vi "test Add Find Remove CD.vi"(8 "error in (no error)":errorcluster, 11 "TestCase in":refnum<class "Embedded Data Logger Scripting Unit Tests.lvclass">) -> (0 "error out":errorcluster, 3 "TestCase out":refnum<class "Embedded Data Logger Scripting Unit Tests.lvclass">)   [LabVIEW 2027, in "Embedded Data Logger Scripting Unit Tests.lvclass"]
uses:
  Embedded Data Logger Scripting Unit Tests.lvclass
  C:/Program Files/National Instruments/LabVIEW 2027/vi.lib/NI/VeriStand Custom Device Testing Tools/VeriStandScriptingTestCase/VeriStandScriptingTestCase.lvclass
  <vilib>/NI VeriStand/Custom Device API/Custom Device Item Ref.ctl
  <vilib>/NI/VeriStand Custom Device Testing Tools/VeriStandScriptingTestCase/VeriStandScriptingTestCase.lvclass/VeriStandScriptingTestCase.ctl
  <vilib>/NI/VeriStand Custom Device Testing Tools/VeriStandScriptingTestCase/Read Target.vi
  C:/NetCoreDLL/NationalInstruments.VeriStand.SystemDefinitionAPI.dll
  NetCoreDLL/NationalInstruments.VeriStand.SystemDefinitionAPI.dll
  C:/Program Files/National Instruments/LabVIEW 2027/vi.lib/addons/_JKI Toolkits/VI Tester/TestCase.llb/TestCase.lvclass
  <vilib>/addons/_JKI Toolkits/VI Tester/TestCase.llb/TestCase.lvclass
  Embedded Data Logger Scripting.lvlib
  <vilib>/NI VeriStand/Custom Device API/Custom Device API.lvlib
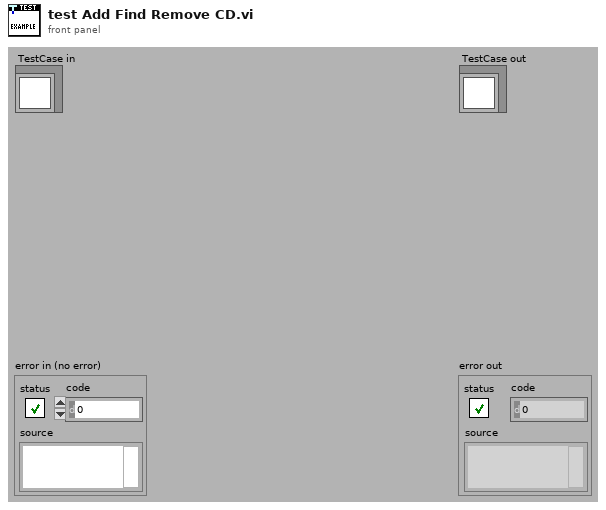
[diagram p1: front panel]
types:
  T1 = typedef "Custom Device API.lvlib/Custom Device Item Ref.ctl" = u64
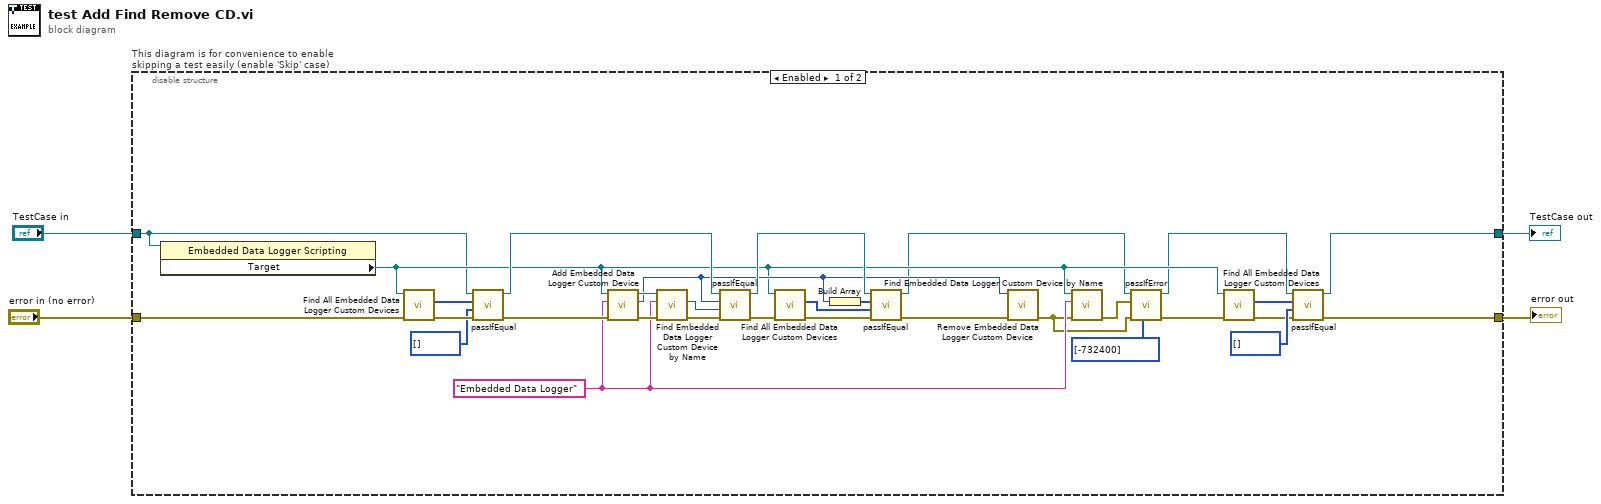
[diagram p0: block diagram]
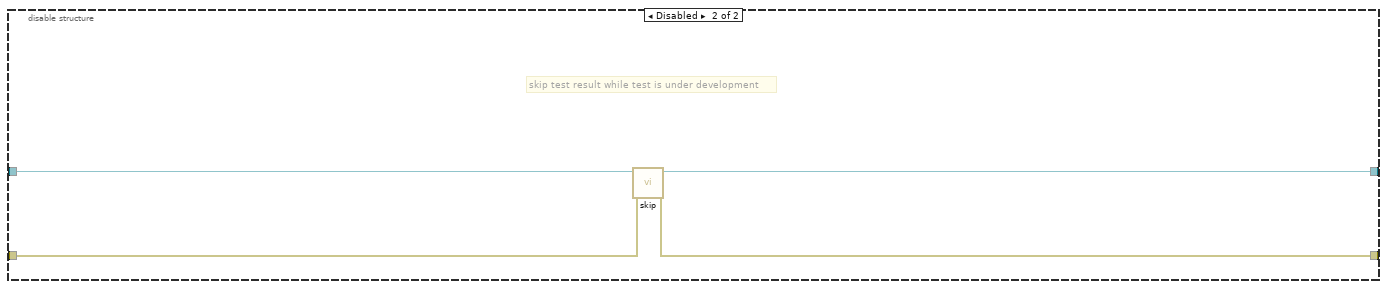
[diagram p2: hidden frame]
diagram:
  n1 = disable-structure "This diagram is for convenience to enable skipping a test easily (enable 'Skip' case)" shown="Enabled" {
    disable-tunnel: "TestCase in" -> [w5 w39]
    disable-tunnel: [w14 w37] -> w1
    disable-tunnel: [w15 w38] -> w3
    disable-tunnel: "error in (no error)" -> [w35 w36]
    frame Enabled {
      w12 = "Embedded Data Logger" ("name")
      n2 = property class="Embedded Data Logger Scripting "(reference=w5) -> ("Target"=w13:refnum<k39>)  [unwired: 1 in, 2 out]
      n3 = call "Find All Embedded Data Logger Custom Devices.vi"("error in"=w35, "NationalInstruments.VeriStand.SystemDefinitionAPI.Target"=w13) -> ("error out"=w34:errorcluster, "embedded data loggers"=w32:T1[])  [unwired: 7 in, 1 out]
      n4 = call-dynamic "passIfEqual.vi"("error in (no error)"=w34, "y"=T1[] [] ("embedded data logger custom devices"), "x"=w32, "TestCase in"=w5) -> ("error out"=w33:errorcluster, "TestCase out"=w23:refnum<class "Embedded Data Logger Scripting Unit Tests.lvclass">)  [unwired: 6 in]
      n5 = call "Add Embedded Data Logger Custom Device.vi"("error in"=w33, "name"=w12, "NationalInstruments.VeriStand.SystemDefinitionAPI.Target"=w13) -> ("error out"=w30:errorcluster, "embedded data logger"=w19:T1, "NationalInstruments.VeriStand.SystemDefinitionAPI.Target"=w29:refnum<k39>)  [unwired: 6 in]
      n6 = call "Find Embedded Data Logger Custom Device by Name.vi"("error in"=w30, "name"=w12, "NationalInstruments.VeriStand.SystemDefinitionAPI.Target"=w29) -> ("error out"=w26:errorcluster, "embedded data logger"=w24:T1)  [unwired: 6 in, 1 out]
      n7 = call-dynamic "passIfEqual.vi"("error in (no error)"=w26, "y"=w24, "x"=w19, "TestCase in"=w23) -> ("error out"=w25:errorcluster, "TestCase out"=w22:refnum<class "Embedded Data Logger Scripting Unit Tests.lvclass">)  [unwired: 6 in]
      n8 = call "Find All Embedded Data Logger Custom Devices.vi"("error in"=w25, "NationalInstruments.VeriStand.SystemDefinitionAPI.Target"=w13) -> ("error out"=w28:errorcluster, "embedded data loggers"=w21:T1[])  [unwired: 7 in, 1 out]
      n9 = Build Array(w19) -> (w20:T1[])
      n10 = call-dynamic "passIfEqual.vi"("error in (no error)"=w28, "y"=w21, "x"=w20, "TestCase in"=w22) -> ("error out"=w27:errorcluster, "TestCase out"=w9:refnum<class "Embedded Data Logger Scripting Unit Tests.lvclass">)  [unwired: 6 in]
      n11 = call "Remove Embedded Data Logger Custom Device.vi"("error in"=w27, "embedded data logger custom device"=w19) -> ("error out"=w11:errorcluster)  [unwired: 9 in]
      n12 = call "Find Embedded Data Logger Custom Device by Name.vi"("error in"=w11, "name"=w12, "NationalInstruments.VeriStand.SystemDefinitionAPI.Target"=w13) -> ("error out"=w10:errorcluster)  [unwired: 6 in, 2 out]
      n13 = call-dynamic "passIfError.vi"("passing error codes (default = any error code)"=i32[] [-732400], "error in (no error)"=w11, "error"=w10, "TestCase in"=w9) -> ("error out"=w7:errorcluster, "TestCase out"=w8:refnum<class "Embedded Data Logger Scripting Unit Tests.lvclass">)  [unwired: 6 in]
      n14 = call "Find All Embedded Data Logger Custom Devices.vi"("error in"=w7, "NationalInstruments.VeriStand.SystemDefinitionAPI.Target"=w13) -> ("error out"=w16:errorcluster, "embedded data loggers"=w17:T1[])  [unwired: 7 in, 1 out]
      n15 = call-dynamic "passIfEqual.vi"("error in (no error)"=w16, "y"=T1[] [] ("embedded data logger custom devices"), "x"=w17, "TestCase in"=w8) -> ("error out"=w15:errorcluster, "TestCase out"=w14:refnum<class "Embedded Data Logger Scripting Unit Tests.lvclass">)  [unwired: 6 in]
    }
    frame Disabled {
      # "skip test result while test is under development"
      n16 = call <vilib>:"skip.vi"("error in (no error)"=w36, "TestCase in"=w39) -> ("error out"=w38:errorcluster, "TestCase out"=w37:refnum<class "Embedded Data Logger Scripting Unit Tests.lvclass">)  [unwired: 8 in]
    }
  }
  "error out" <- w3
  "TestCase out" <- w1
